vi "repeat cycle_exponential up.vi"(8 "error in (no error)":errorcluster caption="에러 입력(에러 없음)", 10 "waveform in":waveform(dbl), 11 "Waveform Obj 입력":refnum<class "Waveform Gen.lvclass">) -> (0 "error out":errorcluster caption="에러 출력", 2 "waveform out":waveform(dbl), 3 "Waveform Obj 출력":refnum<class "Waveform Gen.lvclass">)   [LabVIEW 2020, in "Waveform Gen.lvclass"]
uses:
  Waveform Gen.lvclass
  Waveform Gen.lvclass/Waveform Gen.ctl
  Accessors/Read cycle.vi
  <vilib>/Waveform/WDTOps.llb/WDT Append Waveforms DBL.vi
  <vilib>/Waveform/WDTOps.llb/WDT Number of Waveform Samples DBL.vi
  <vilib>/Waveform/WDTOps.llb/WDT Get Waveform Subset DBL.vi
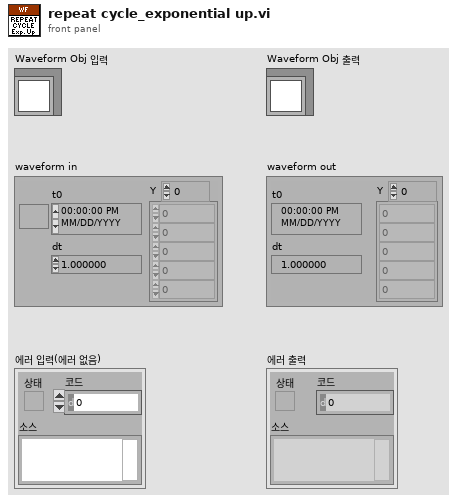
[diagram p1: front panel]
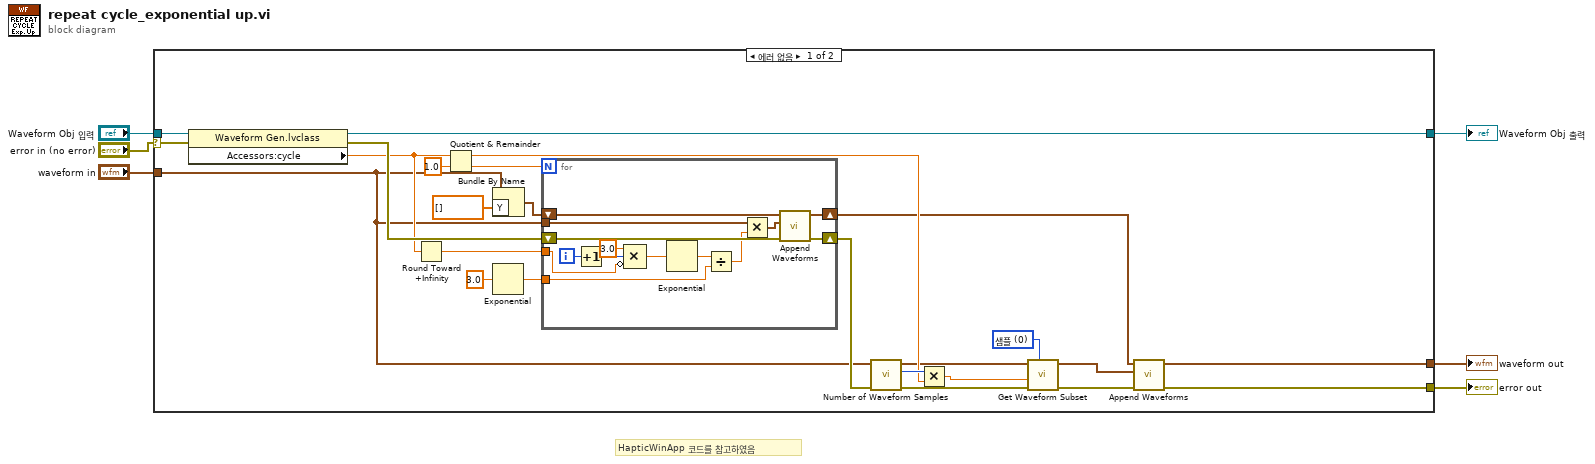
[diagram p0: block diagram]
diagram:
  # "HapticWinApp 코드를 참고하였음"
  n1 = case shown="에러 없음" "error in (no error)" {
    selector: "error in (no error)" -> [w29 w47]
    tunnel: [w8 w47] -> w3
    tunnel: "Waveform Obj 입력" -> [w31 w46]
    tunnel: [w9 w46] -> w5
    tunnel: "waveform in" -> [w10 _]
    tunnel: [w7 _] -> w1
    frame No Error {
      w19 = u16 0 items=["샘플", "상대 시간"] ("start/duration format")
      n2 = property class="Waveform Gen.lvclass"(reference=w31, error in=w29) -> (reference out=w9:refnum<class "Waveform Gen.lvclass">, error out=w22:errorcluster, "Accessors:cycle"=w18:dbl)
      n3 = Round Toward +Infinity(x=w18) -> (ceil(x): smallest int >= x=w16:dbl)
      n4 = Quotient & Remainder(x=w18, y=1.0) -> (x-y*floor(x/y)=w26:dbl, floor(x/y)=w28:dbl)
      n5 = Bundle By Name(cluster=w10, "Y"=dbl[] []) -> (w12:waveform(dbl))
      n6 = Exponential(1:3.0 ("x")) -> (0:w15:dbl)
      n7 = for {
        N: w28 -> [_]
        shift-right: [w44] -> w13
        shift-left: w12 -> [w45]
        shift-right: [w42] -> w21
        shift-left: w22 -> [w43]
        tunnel: w10 -> [w41]
        tunnel: w16 -> [w36]
        tunnel: w15 -> [w33]
        i -> [w40]
        n8 = Increment(x=w40) -> (x+1=w38:i32)
        n9 = Compound Arithmetic op=MULTIPLY(3.0 ("값"), w38, invert w36) -> (w35:dbl)
        n10 = Exponential(1:w35) -> (0:w34:dbl)
        n11 = Divide(x=w34, y=w33) -> (x/y=w32:dbl)
        n12 = Multiply(x=w41, y=w32) -> (x*y=w39:waveform(dbl))
        n13 = call-poly <vilib>:"Append Waveforms.vi"("error in (no error)"=w43, "waveform B"=w39, "waveform A"=w45) -> ("error out"=w42:errorcluster, "waveform out"=w44:waveform(dbl))  [unwired: 7 in]
      }
      n14 = call-poly <vilib>:"Number of Waveform Samples.vi"("error in (no error)"=w21, "waveform in"=w10) -> ("error out"=w24:errorcluster, "number of samples"=w27:i32, "waveform out"=w14:waveform(dbl))  [unwired: 7 in]
      n15 = Multiply(x=w27, y=w26) -> (x*y=w25:dbl)
      n16 = call-poly <vilib>:"Get Waveform Subset.vi"("start/duration format"=w19, "error in (no error)"=w24, "duration"=w25, "waveform in"=w14) -> ("error out"=w20:errorcluster, "waveform out"=w23:waveform(dbl))  [unwired: 2 in, 2 out]
      n17 = call-poly <vilib>:"Append Waveforms.vi"("error in (no error)"=w20, "waveform B"=w23, "waveform A"=w13) -> ("error out"=w8:errorcluster, "waveform out"=w7:waveform(dbl))  [unwired: 7 in]
    }
    frame Error {
    }
  }
  "error out" <- w3
  "Waveform Obj 출력" <- w5
  "waveform out" <- w1
